vi "ATF-Pump-AI_Read.vi"(5 "Data FIFO Ref":T1, 6 "error in (no error)":errorcluster, 7 "Numeric":dbl=10.0, 9 "AI_Task":refnum<k21>) -> (0 "error out":errorcluster, 3 "task out":refnum<k21>)   [LabVIEW 2022 SP3]
uses:
  RT Controls/ATF-Pump-Data FIFO.ctl
  <vilib>/DAQmx/read.llb/DAQmx Read (Analog 1D Wfm NChan NSamp).vi
  <vilib>/DAQmx/miscellaneous.llb/DAQmx Fill In Error Info.vi
panel:
  out "overflow?":bool
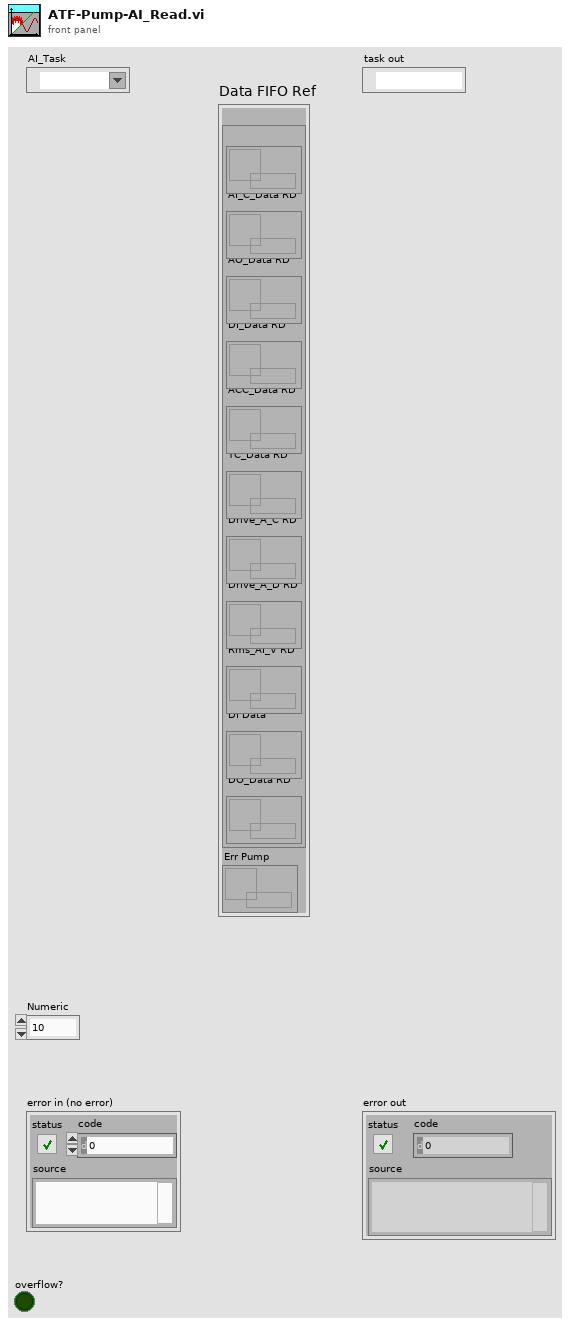
[diagram p1: front panel]
types:
  T1 = typedef "ATF-Pump-Data FIFO.ctl" = cluster{"RD":cluster{"AI_V_Data RD":refnum<queue>, "AI_C_Data RD":refnum<queue>, "AO_Data RD":refnum<queue>, "DI_Data RD":refnum<queue>, "ACC_Data RD":refnum<queue>, "TC_Data RD":refnum<queue>, "Drive_A_C RD":refnum<queue>, "Drive_A_D RD":refnum<queue>, "Rms_AI_V RD":refnum<queue>, "DI Data":refnum<queue>, "DO_Data RD":refnum<queue>}, "Err Pump":refnum<queue>}
  T2 = enum16{"AI C", "AI V", "AO", "DI", "DO", "TC", "ACC", "RT PMP", "DR A"}
  T3 = enum16{"Init", "Read 'All'", "Read 'n'", "Read '1'", "Write '1'", "Write 'n'", "Write 'All'"}
  T4 = cluster{"Start DAQ":bool, "Stop DAQ":bool, "RT Stop":bool, "RT Exit":bool, "Start Seq":bool}
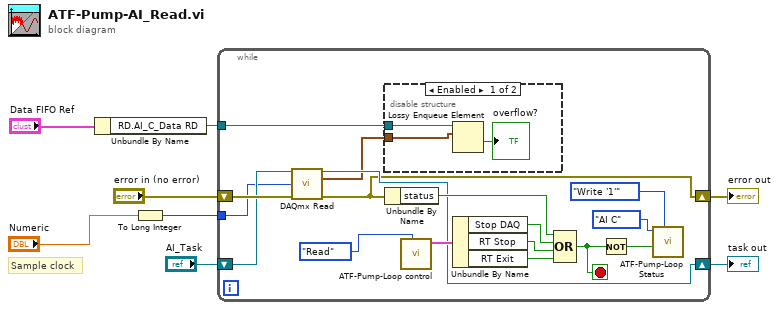
[diagram p0: block diagram]
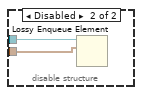
[diagram p2: hidden frame]
diagram:
  # "Sample clock"
  n1 = Unbundle By Name("Data FIFO Ref") -> ("RD.AI_C_Data RD"=w1:refnum<queue>)
  n2 = To Long Integer(number="Numeric") -> (32bit integer=w5:i32)
  n3 = while {
    tunnel: w5 -> [w9]
    shift-right: [w14] -> w4
    shift-left: "AI_Task" -> [w24]
    shift-right: [w11] -> w3
    shift-left: "error in (no error)" -> [w25]
    tunnel: w1 -> [w13]
    stop <- w23 stop-if-true
    n4 = call-poly <vilib>:"DAQmx Read.vi"("task/channels in"=w24, "number of samples per channel"=w9, "error in"=w25) -> ("task out"=w14:refnum<k21>, "data"=w12:waveform(dbl)[], "error out"=w11:errorcluster)  [unwired: 10 in]
    n5 = disable-structure shown="Enabled" {
      disable-tunnel: w13 -> [w28 w30]
      disable-tunnel: w12 -> [w27 w29]
      frame Enabled {
        n6 = Lossy Enqueue Element(queue=w28, element=w27) -> (overflow?=→"overflow?":bool)  [unwired: 1 in, 3 out]
      }
      frame Disabled {
        n7 = Lossy Enqueue Element(queue=w30, element=w29) -> ()  [unwired: 1 in, 4 out]
      }
    }
    n8 = Unbundle By Name(w11) -> ("status"=w22:bool)
    n9 = call "ATF-Pump-Loop control.vi"("Action"=enum16{"Init", "Write", "Read"}."Read") -> ("Loop Control out"=w21:T4)  [unwired: 9 in, 1 out]
    n10 = Unbundle By Name(w21) -> ("Stop DAQ"=w20:bool, "RT Stop"=w19:bool, "RT Exit"=w18:bool)
    n11 = Compound Arithmetic op=OR(w22, w20, w19, w18) -> (w23:bool)
    n12 = Not(x=w23) -> (.not. x?=w15:bool)
    n13 = call "ATF-Pump-Loop Status.vi"("Option"=T3."Write '1'", "Status"=w15, "Loop"=T2."AI C") -> ()  [unwired: 6 in, 3 out]
  }
  "task out" <- w4
  "error out" <- w3
